vi "SimpleTest.vi"() -> ()   [LabVIEW 2014]
panel:
  out "Inherent IVI Settings:Instrument Identification:Model":string
  in  "btnAbortGen":bool
  in  "BtnInitGen":bool
  in  "reset device":bool=TRUE caption="reset device (True)"
  in  "btnGetProperties":bool
  in  "btnClose":bool
  in  "IVI Logical Name":refnum<k15>
  in  "btnOpen":bool
  in  "Stop Button":bool
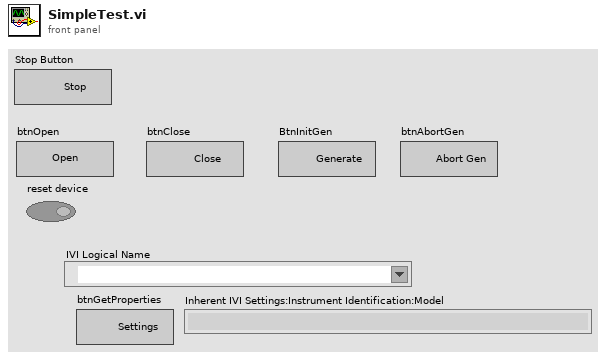
[diagram p1: front panel]
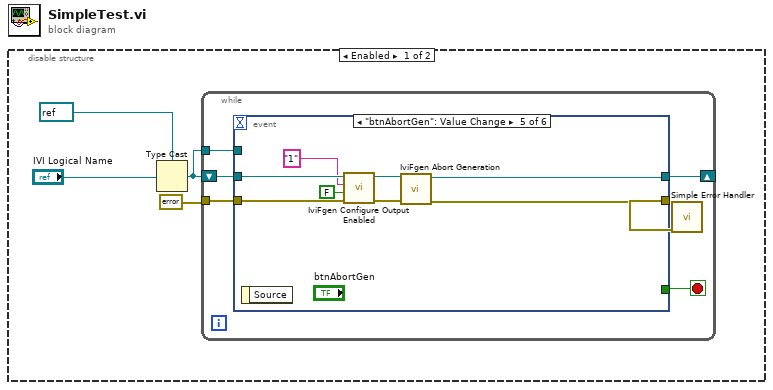
[diagram p0: block diagram]
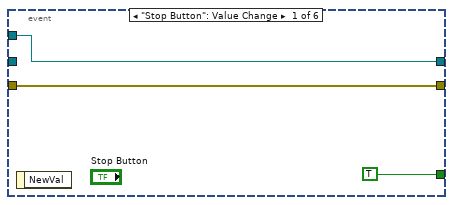
[diagram p2: hidden frame]
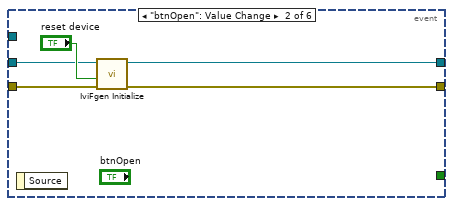
[diagram p3: hidden frame]
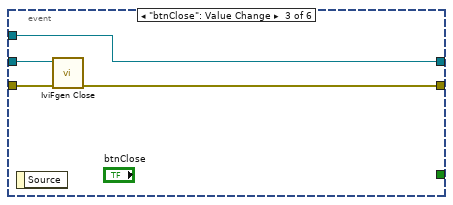
[diagram p4: hidden frame]
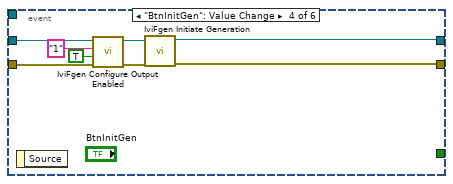
[diagram p5: hidden frame]
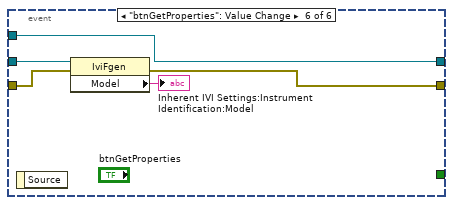
[diagram p6: hidden frame]
diagram:
  n1 = disable-structure shown="Enabled" {
    frame Enabled {
      n2 = Type Cast(type=refnum<k15> refnum ("logical name (\"SampleDmm\")"), x="IVI Logical Name") -> (*(type *) &x=w1:refnum<k15>)
      n3 = while {
        shift-right: [w6] -> _
        shift-left: w1 -> [w5]
        tunnel: errorcluster {"status"=FALSE, "code"=0, "source"=""} ("error in (no error)") -> [w9]
        tunnel: w1 -> [w8]
        stop <- w10 stop-if-true
        n4 = event shown="[4] \"btnAbortGen\": Value Change" {
          selector: _ -> [_ _ _ _ _ _]
          dyn-events: _ -> [_ _ _ _ _ _]
          timeout: _ -> [_ _ _ _ _ _]
          tunnel: [TRUE _ _ _ _ _] -> w10
          tunnel: w9 -> [w12 w18 w22 w28 w36 w43]
          tunnel: [w12 w17 w21 w29 w37 w42] -> w7
          tunnel: w8 -> [w11 _ w19 _ _ w39]
          tunnel: [w11 w15 w19 w30 w38 w39] -> w6
          tunnel: w5 -> [_ w14 w20 w26 w35 w41]
          event "Stop Button": Value Change {
            n5 = event-data() -> ()  [unwired: 1 in, 1 out]
          }
          event "btnOpen": Value Change {
            n6 = event-data() -> ()  [unwired: 1 in, 1 out]
            n7 = call <vilib>:"IviFgen Initialize.vi"("error in (no error)"=w18, "reset device (true)"="reset device", "logical name (\"SampleFGen\")"=w14) -> ("error out"=w17:errorcluster, "instrument handle out"=w15:refnum<k15>)  [unwired: 7 in]
          }
          event "btnClose": Value Change {
            n8 = event-data() -> ()  [unwired: 1 in, 1 out]
            n9 = call <vilib>:"IviFgen Close.vi"("error in (no error)"=w22, "instrument handle"=w20) -> ("error out"=w21:errorcluster)  [unwired: 9 in]
          }
          event "BtnInitGen": Value Change {
            n10 = event-data() -> ()  [unwired: 1 in, 1 out]
            n11 = call <vilib>:"IviFgen Configure Output Enabled.vi"("error in (no error)"=w28, "channel enabled (True)"=TRUE, "channel name (\"CHANNEL1\")"="1" ("channel name (\"CHANNEL1\")"), "instrument handle"=w26) -> ("error out"=w27:errorcluster, "instrument handle out"=w25:refnum<k15>)  [unwired: 6 in]
            n12 = call <vilib>:"IviFgen Initiate Generation.vi"("error in (no error)"=w27, "instrument handle"=w25) -> ("error out"=w29:errorcluster, "instrument handle out"=w30:refnum<k15>)  [unwired: 8 in]
          }
          event "btnAbortGen": Value Change {
            n13 = event-data() -> ()  [unwired: 1 in, 1 out]
            n14 = call <vilib>:"IviFgen Configure Output Enabled.vi"("error in (no error)"=w36, "channel enabled (True)"=FALSE, "channel name (\"CHANNEL1\")"="1", "instrument handle"=w35) -> ("error out"=w32:errorcluster, "instrument handle out"=w31:refnum<k15>)  [unwired: 6 in]
            n15 = call <vilib>:"IviFgen Abort Generation.vi"("error in (no error)"=w32, "instrument handle"=w31) -> ("error out"=w37:errorcluster, "instrument handle out"=w38:refnum<k15>)  [unwired: 8 in]
          }
          event "btnGetProperties": Value Change {
            n16 = event-data() -> ()  [unwired: 1 in, 1 out]
            n17 = property class="IviFgen"(reference=w41, error in=w43) -> (error out=w42:errorcluster, "Model"=→"Inherent IVI Settings:Instrument Identification:Model":string)  [unwired: 1 out]
          }
        }
        n18 = call <vilib>:"Simple Error Handler.vi"("error in (no error)"=w7) -> ()  [unwired: 4 in, 5 out]
      }
    }
    frame Disabled {
    }
  }
